vi "Log MBW Data.vi"() -> ()   [LabVIEW 2015]
uses:
  X Range.ctl
  MBW States.ctl
  <vilib>/Instr/_visa.llb/VISA Configure Serial Port (Instr).vi
  <vilib>/Utility/file.llb/Write To Spreadsheet File (string).vi
panel:
  out "Cycle Time, ms":u32=618
  out "Ch3":sgl=35854.33
  out "Ch2":sgl=35854.33
  out "Ch1":sgl=35854.33
  out "Ch0":sgl=26047.0
  in  "Re-Initialize":bool
  out "error out":errorcluster
  in  "States":T1=enum."Initialize"
  in  "CH D":u16(ring) items=["Time_s", "Stable", "Frostpoint_C", "DewPoint_C", "VolRatio_ppmv", "VaporPres_Pa", "HeadPres_Pa", "FlowRate_lpm", "MirrorT_C"]
  in  "CH C":u16(ring) items=["Time_s", "Stable", "Frostpoint_C", "DewPoint_C", "VolRatio_ppmv", "VaporPres_Pa", "HeadPres_Pa", "FlowRate_lpm", "MirrorT_C"]
  in  "CH B":u16(ring) items=["Time_s", "Stable", "Frostpoint_C", "DewPoint_C", "VolRatio_ppmv", "VaporPres_Pa", "HeadPres_Pa", "FlowRate_lpm", "MirrorT_C"]
  in  "CH A":u16(ring)=4 items=["Time_s", "Stable", "Frostpoint_C", "DewPoint_C", "VolRatio_ppmv", "VaporPres_Pa", "HeadPres_Pa", "FlowRate_lpm", "MirrorT_C"]
  out "Graph 2":sgl[][](graph)=[[35846.125, 35846.75, 35847.375, 35848.016, 35848.688, 35849.297, 35849.92, 35850.53, 35851.14, 35851.766, 35852.375, 35853.03, 35853.703], [35846.125, 35846.75, 35847.375, 35848.016, 35848.688, 35849.297, 35849.92, 35850.53, 35851.14, 35851.766, 35852.375, 35853.03, 35853.703]]
  out "Graph 1":sgl[][](graph)=[[25759.9, 25973.8, 25975.8, 25975.8, 25980.7, 25987.2, 25987.2, 25998.8, 25998.8, 26008.6, 26020.1, 26020.1, 26032.8], [35846.125, 35846.75, 35847.375, 35848.016, 35848.688, 35849.297, 35849.92, 35850.53, 35851.14, 35851.766, 35852.375, 35853.03, 35853.703]]
  in  "X Range":T2
  out "Current File":path=path "C:/MBW_Data/MBW20120124/MBW20120124x003.txt"
  in  "Base Path":path=path "C:/MBW_Data"
  in  "stop":bool
  in  "Column Header (comma del)":string="Time_s,Stable,Frostpoint_C,DewPoint_C,VolRatio_ppmv,VaporPres_Pa,HeadPres_Pa,FlowRate_lpm,MirrorT_C"
  in  "Sample rate (S)":u32=1
  in  "Commands to send":string[](array[string])=["Stable?", "FP?", "DP?", "PPMv?", "VP?", "P?", "Flow?", "Tm?"]
  in  "Com Port":refnum<visa-resource-name>="COM4"
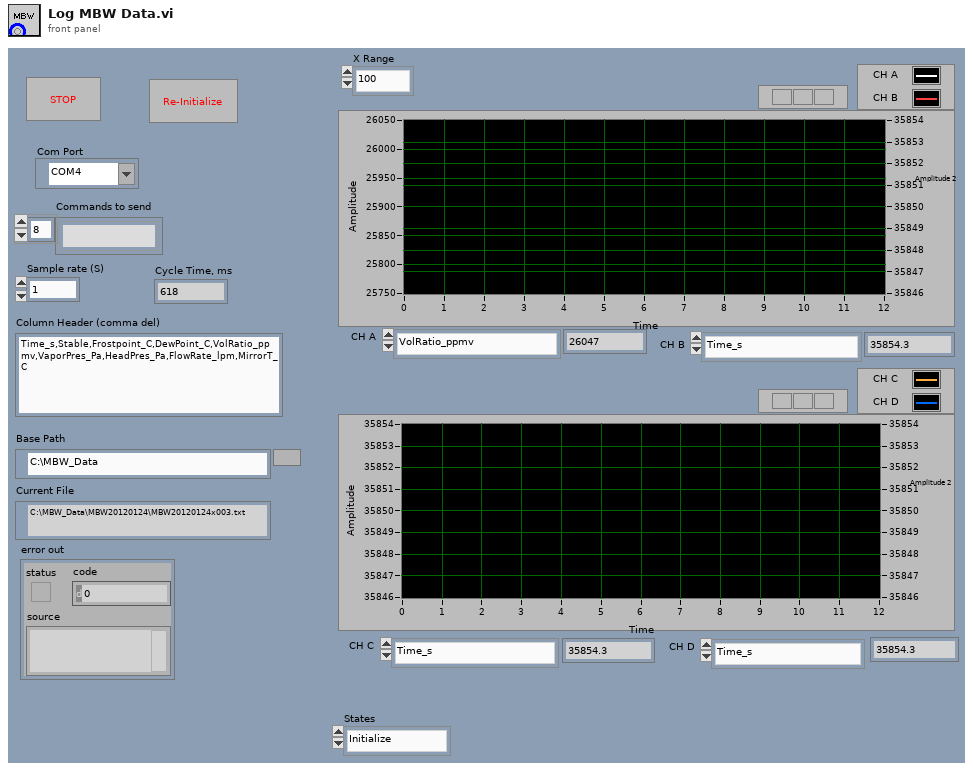
[diagram p1: front panel]
types:
  T1 = typedef "MBW States.ctl" = enum16{"Idle", "Initialize", "Check Buttons", "Send Commands", "Update Graph", "Write Data", "Close", "Exit"}
  T2 = typedef "X Range.ctl" = enum16{"100", "300", "500", "1000", "3000", "5000", "10000", "20000", "30000", "40000", "60000"}
  T3 = typedef "LVDateTimeRec.ctl" = cluster{"fractional second":dbl, "second":i32, "minute":i32, "hour":i32, "day of month":i32, "month":i32, "year":i32, "day of week":i32, "day of year":i32, "DST":i32}
  T4 = cluster{"CH A":u16, "CH B":u16, "CH C":u16, "CH D":u16}
  T5 = cluster{"Ch0":sgl, "Ch1":sgl, "Ch2":sgl, "Ch3":sgl}
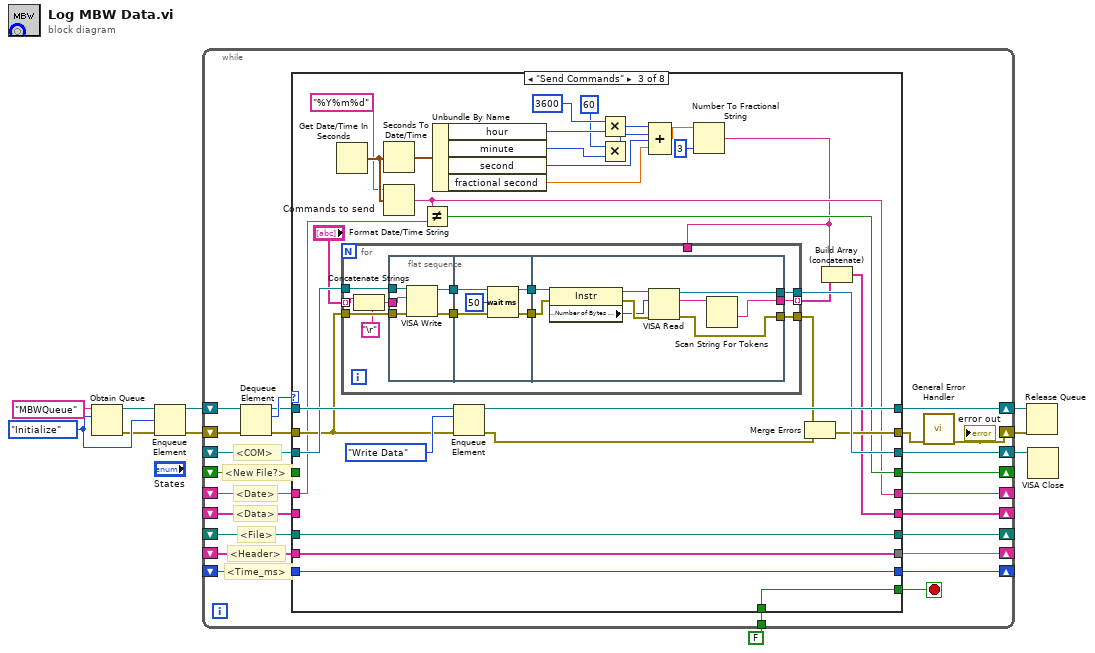
[diagram p0: block diagram]
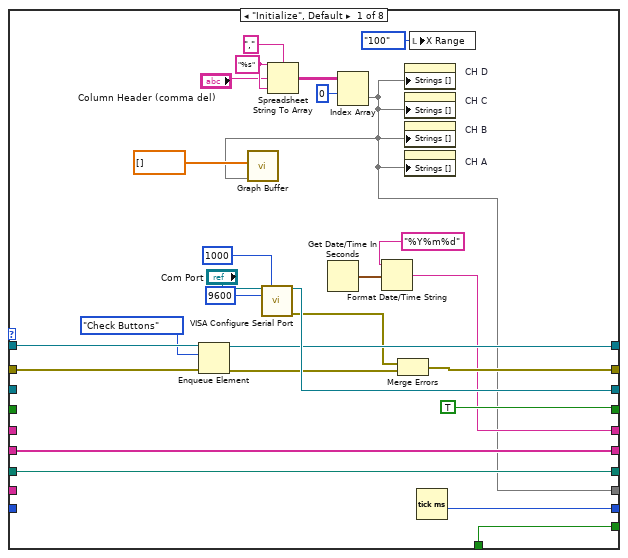
[diagram p2: hidden frame]
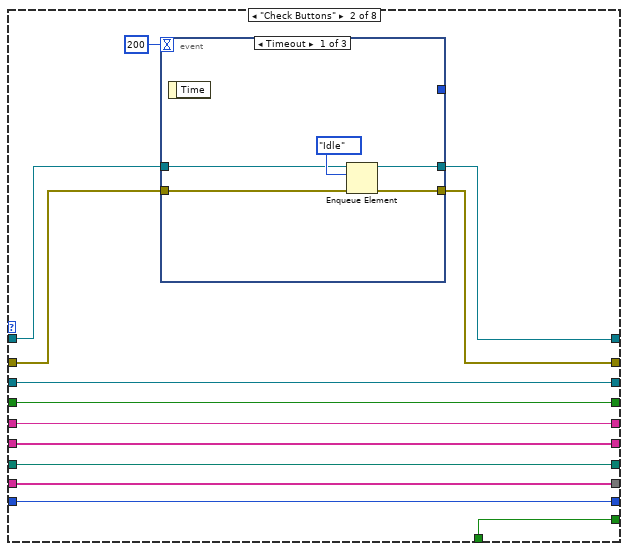
[diagram p3: hidden frame]
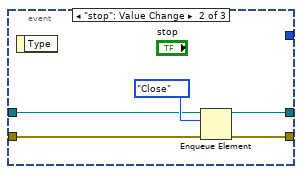
[diagram p4: hidden frame]
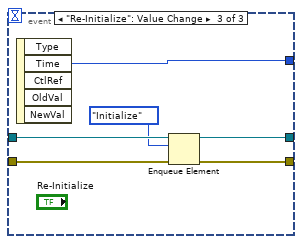
[diagram p5: hidden frame]
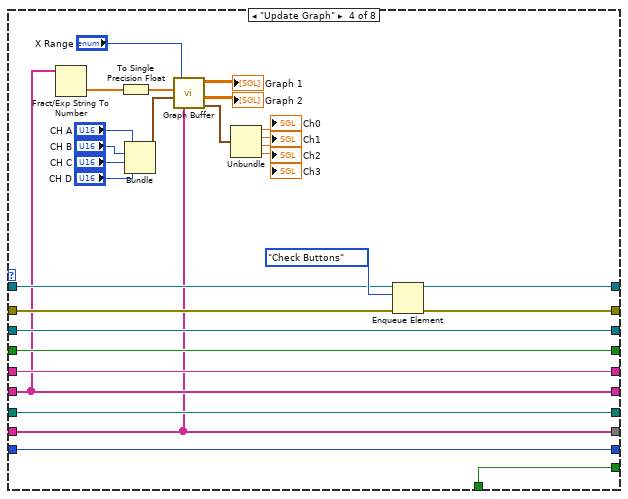
[diagram p6: hidden frame]
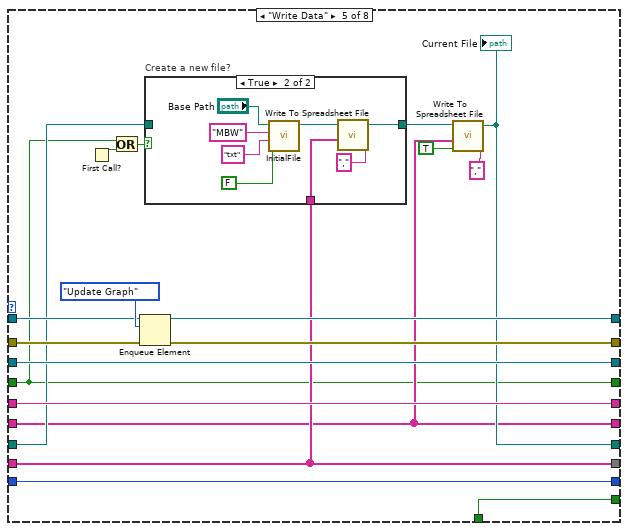
[diagram p7: hidden frame]
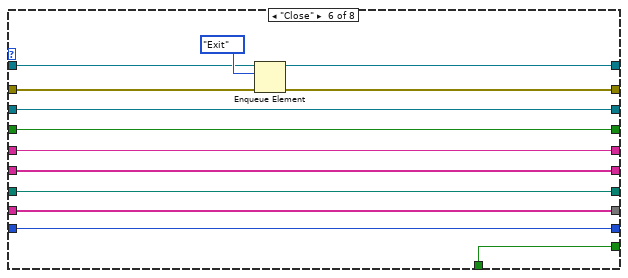
[diagram p9: hidden frame]
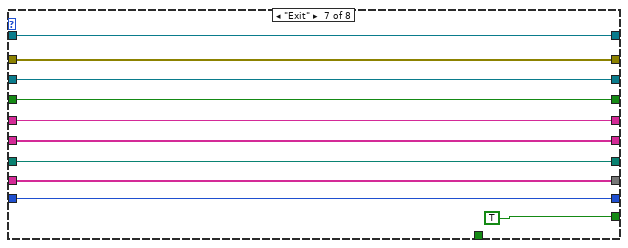
[diagram p10: hidden frame]
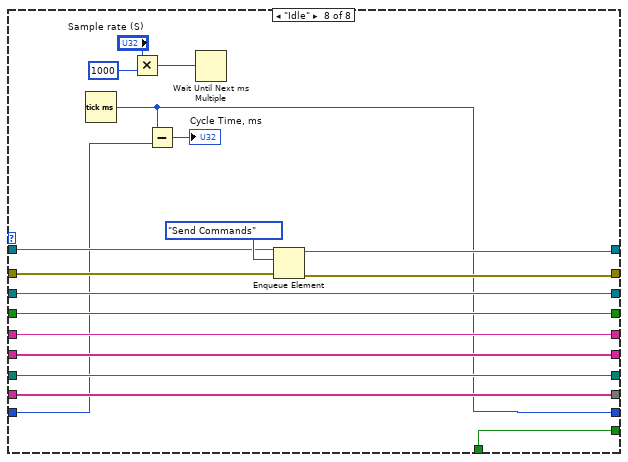
[diagram p11: hidden frame]
diagram:
  w9 = MBW_States."Initialize" ("States")
  n1 = Obtain Queue(name (unnamed)="MBWQueue", element data type=w9) -> (queue out=w8:refnum<queue>, error out=w7:errorcluster)  [unwired: 3 in, 1 out]
  n2 = Enqueue Element(queue=w8, element=w9, error in (no error)=w7) -> (queue out=w6:refnum<queue>, error out=w5:errorcluster)  [unwired: 1 in, 1 out]
  n3 = while {
    shift-right: [w25] -> w4
    shift-left: w6 -> [w28]
    shift-right: [w24] -> w3
    shift-left: w5 -> [w30]
    shift-right: [w33] -> w2
    shift-left: _ -> [w34]
    shift-right: [w31] -> _
    shift-left: _ -> [w32]
    shift-right: [w22] -> _
    shift-left: _ -> [w23]
    shift-right: [w20] -> _
    shift-left: _ -> [w21]
    shift-right: [w18] -> _
    shift-left: _ -> [w19]
    shift-right: [w16] -> _
    shift-left: _ -> [w17]
    tunnel: FALSE -> [w15]
    shift-right: [w12] -> _
    shift-left: _ -> [w13]
    stop <- w14 stop-if-true
    # "<Time_ms>"
    # "<Header>"
    # "<File>"
    # "<Date>"
    # "<Data>"
    # "<New File?>"
    # "<COM>"
    n4 = Dequeue Element(queue=w28, error in (no error)=w30) -> (queue out=w26:refnum<queue>, element=w27:T1, error out=w29:errorcluster)  [unwired: 1 in, 1 out]
    n5 = case shown="\"Send Commands\"" w27 {
      tunnel: w29 -> [w47 w71 w108 w174 w195 w211 w231 w236]
      tunnel: [w49 w68 w105 w173 w194 w210 w231 w237] -> w11
      tunnel: w34 -> [_ w74 w111 w180 w199 w221 w230 w249]
      tunnel: [w60 w74 w110 w180 w199 w221 w230 w249] -> w33
      tunnel: w32 -> [_ w73 _ w179 w183 w220 w229 w248]
      tunnel: [TRUE w73 w98 w179 w183 w220 w229 w248] -> w31
      tunnel: w26 -> [w48 w72 w122 w176 w197 w213 w228 w239]
      tunnel: [w52 w67 w121 w175 w196 w212 w228 w238] -> w25
      tunnel: w23 -> [_ w70 w99 w178 w193 w219 w227 w247]
      tunnel: [w41 w70 w97 w178 w193 w219 w227 w247] -> w22
      tunnel: w21 -> [w45 w69 _ w169 w188 w218 w226 w246]
      tunnel: [w45 w69 w101 w169 w188 w218 w226 w246] -> w20
      tunnel: w19 -> [w40 w66 w96 w172 w191 w217 w225 w245]
      tunnel: [w40 w66 w96 w172 w189 w217 w225 w245] -> w18
      tunnel: w17 -> [_ w65 w95 w161 w190 w216 w224 w244]
      tunnel: [w35 w65 w95 w161 w190 w216 w224 w244] -> w16
      tunnel: w15 -> [w39 w64 w94 w171 w186 w215 _ w243]
      tunnel: [w39 w64 w94 w171 w186 w215 TRUE w243] -> w14
      tunnel: w13 -> [_ w62 w92 w170 w185 w209 w222 w234]
      tunnel: [w38 w62 w92 w170 w185 w209 w222 w233] -> w12
      frame "Initialize", Default {
        w58 = "%s" ("format string")
        n6 = Enqueue Element(queue=w48, element=MBW_States."Check Buttons", error in (no error)=w47) -> (queue out=w52:refnum<queue>, error out=w50:errorcluster)  [unwired: 1 in, 1 out]
        n7 = call-poly "VISA Configure Serial Port"("VISA resource name"="Com Port", "timeout (10sec)"=u32 1000, "baud rate (9600)"=u32 9600) -> ("VISA resource name out"=w60:refnum<visa-resource-name>, "error out"=w51:errorcluster)  [unwired: 11 in]
        n8 = Spreadsheet String To Array(delimiter (Tab)=",", format string=w58, spreadsheet string="Column Header (comma del)", array type (2D Dbl)=w58) -> (array=w36:string[][])
        n9 = Get Date/Time In Seconds() -> (seconds since 1Jan1904=w42:timestamp)
        n10 = Index Array(array=w36, index (row)=0) -> (element=w35:string[])  [unwired: 1 in]
        n11 = call "Graph Buffer.vi"("Channel Names"=w35, "Data"=sgl[] []) -> ()  [unwired: 3 in, 3 out]
        n12 = Format Date/Time String(time format string (%c)="%Y%m%d", seconds (now)=w42) -> (date/time string=w41:string)  [unwired: 1 in]
        n13 = Merge Errors(w51, w50) -> (w49:errorcluster)
        n14 = property on="CH D" class="Ring (strict)"("Strings []"=w35) -> ()  [unwired: 2 in, 2 out]
        n15 = property on="CH C" class="Ring (strict)"("Strings []"=w35) -> ()  [unwired: 2 in, 2 out]
        n16 = property on="CH B" class="Ring (strict)"("Strings []"=w35) -> ()  [unwired: 2 in, 2 out]
        n17 = property on="CH A" class="Ring (strict)"("Strings []"=w35) -> ()  [unwired: 2 in, 2 out]
        n18 = local write "X Range"(X_Range."100" ("X Range")) -> ()
        n19 = Tick Count (ms)() -> (millisecond timer value=w38:u32)
      }
      frame "Check Buttons" {
        n20 = event shown="[0] Timeout" {
          selector: _ -> [_ _ _]
          dyn-events: _ -> [_ _ _]
          timeout: 200 -> [_ _ _]
          tunnel: w72 -> [w76 w83 w90]
          tunnel: w71 -> [w75 w81 w89]
          tunnel: [w77 w80 w88] -> w68
          tunnel: [w78 w82 w87] -> w67
          tunnel: [_ _ w85] -> _
          event Timeout {
            n21 = event-data() -> ()  [unwired: 1 in, 1 out]
            n22 = Enqueue Element(queue=w76, element=MBW_States."Idle", error in (no error)=w75) -> (queue out=w78:refnum<queue>, error out=w77:errorcluster)  [unwired: 1 in, 1 out]
          }
          event "stop": Value Change {
            n23 = event-data() -> ()  [unwired: 1 in, 1 out]
            n24 = Enqueue Element(queue=w83, element=MBW_States."Close", error in (no error)=w81) -> (queue out=w82:refnum<queue>, error out=w80:errorcluster)  [unwired: 1 in, 1 out]
          }
          event "Re-Initialize": Value Change {
            n25 = event-data() -> ("Time"=w85:u32)  [unwired: 1 in, 4 out]
            n26 = Enqueue Element(queue=w90, element=MBW_States."Initialize", error in (no error)=w89) -> (queue out=w87:refnum<queue>, error out=w88:errorcluster)  [unwired: 1 in, 1 out]
          }
        }
      }
      frame "Send Commands" {
        n27 = Get Date/Time In Seconds() -> (seconds since 1Jan1904=w100:timestamp)
        n28 = Seconds To Date/Time(time stamp (now)=w100) -> (date time rec=w120:T3)  [unwired: 1 in]
        n29 = Format Date/Time String(time format string (%c)="%Y%m%d", seconds (now)=w100) -> (date/time string=w97:string)  [unwired: 1 in]
        n30 = Not Equal?(x=w97, y=w99) -> (x != y?=w98:bool)
        n31 = Unbundle By Name(w120) -> ("hour"=w119:i32, "minute"=w117:i32, "second"=w113:i32, "fractional second"=w112:dbl)
        n32 = Enqueue Element(queue=w122, element=MBW_States."Write Data", error in (no error)=w108) -> (queue out=w121:refnum<queue>, error out=w107:errorcluster)  [unwired: 1 in, 1 out]
        n33 = Multiply(x=3600, y=w119) -> (x*y=w115:i32)
        n34 = Multiply(x=60, y=w117) -> (x*y=w114:i32)
        n35 = Compound Arithmetic op=ADD(w115, w114, w113, w112) -> (w104:dbl)
        n36 = Number To Fractional String(number=w104, precision (6)=i16 3) -> (F-format string=w93:string)  [unwired: 2 in]
        n37 = for {
          tunnel: w111 -> [w135]
          tunnel: [w132] -> w110
          tunnel: "Commands to send" -> [w126] mode=indexing
          tunnel: [w129] -> w106
          tunnel: w108 -> [w128]
          tunnel: [w127] -> w102 mode=indexing
          tunnel: w93 -> [_]
          n38 = Concatenate Strings(w126, "\r") -> (w125:string)
          n39 = flat-sequence {
            tunnel: w135 -> [w140]
            tunnel: [w139] -> w133
            tunnel: w125 -> [w138]
            tunnel: [w137] -> w130
            tunnel: w128 -> [w136]
            tunnel: [w143] -> w134
            tunnel: w133 -> [w143]
            tunnel: [w142] -> w131
            tunnel: w130 -> [w142]
            tunnel: w134 -> [w152]
            tunnel: [w150] -> w132
            tunnel: w131 -> [w149]
            tunnel: [w144] -> w129
            tunnel: [w145] -> w127
            frame #0 {
              n40 = VISA Write(VISA resource name=w140, write buffer=w138, error in (no error)=w136) -> (VISA resource name out=w139:refnum<visa-resource-name>, error out=w137:errorcluster)  [unwired: 1 out]
            }
            frame #1 {
              n41 = Wait (ms)(milliseconds to wait=u32 50) -> ()  [unwired: 1 out]
            }
            frame #2 {
              n42 = property class="Instr"(reference=w152, error in=w149) -> (reference out=w151:refnum<visa-resource-name>, error out=w148:errorcluster, "Serial Settings:Number of Bytes at Serial Port"=w147:u32)
              n43 = VISA Read(VISA resource name=w151, byte count=w147, error in (no error)=w148) -> (VISA resource name out=w150:refnum<visa-resource-name>, read buffer=w146:string, error out=w144:errorcluster)  [unwired: 1 out]
              n44 = Scan String For Tokens(9:w146) -> (1:w145:string)  [unwired: 5 in, 3 out]
            }
          }
        }
        n45 = Merge Errors(w106, w107) -> (w105:errorcluster)
        n46 = Build Array (concatenate)(w93, w102) -> (w101:string[])
      }
      frame "Update Graph" {
        n47 = Fract/Exp String To Number(string=w169) -> (number=w168:dbl[])  [unwired: 3 in, 1 out]
        n48 = To Single Precision Float(number=w168) -> (single precision float=w153:sgl[])
        n49 = Bundle("CH A"="CH A", "CH B"="CH B", "CH C"="CH C", "CH D"="CH D") -> (w162:T4)  [unwired: 1 in]
        n50 = call "Graph Buffer.vi"("Channel Names"=w161, "Channels"=w162, "Data"=w153, "X Range"="X Range") -> ("LastValues"=w158:T5, "Graph 2"=→"Graph 2":sgl[][], "Graph 1"=→"Graph 1":sgl[][])  [unwired: 1 in]
        n51 = Unbundle(w158) -> ("Ch0"=→"Ch0":sgl, "Ch1"=→"Ch1":sgl, "Ch2"=→"Ch2":sgl, "Ch3"=→"Ch3":sgl)
        n52 = Enqueue Element(queue=w176, element=MBW_States."Check Buttons", error in (no error)=w174) -> (queue out=w175:refnum<queue>, error out=w173:errorcluster)  [unwired: 1 in, 1 out]
      }
      frame "Write Data" {
        n53 = First Call?() -> (First Call?: T/F=w182:bool)
        n54 = Or(x=w183, y=w182) -> (x .or. y?=w181:bool)
        n55 = Enqueue Element(queue=w197, element=MBW_States."Update Graph", error in (no error)=w195) -> (queue out=w196:refnum<queue>, error out=w194:errorcluster)  [unwired: 1 in, 1 out]
        n56 = case "Create a new file?" shown="True" w181 {
          tunnel: [w200 w204] -> w192
          tunnel: w191 -> [w200 _]
          tunnel: w190 -> [_ w202]
          frame False {
          }
          frame True {
            n57 = call "InitialFile.vi"("UTC format"=FALSE, "Extension"="txt", "PreAppend Name"="MBW", "Base Path"="Base Path") -> ("File Path"=w203:path)  [unwired: 7 in]
            n58 = call-poly <vilib>:"Write To Spreadsheet File.vi"("delimiter (\\t)"="," ("delimiter (\\t)"), "1D data"=w202, "file path (dialog if empty)"=w203) -> ("new file path (Not A Path if cancelled)"=w204:path)  [unwired: 5 in]
          }
        }
        n59 = call-poly <vilib>:"Write To Spreadsheet File.vi"("delimiter (\\t)"="," ("delimiter (\\t)"), "append to file? (new file:F)"=TRUE, "1D data"=w188, "file path (dialog if empty)"=w192) -> ("new file path (Not A Path if cancelled)"=w189:path)  [unwired: 4 in]
        "Current File" <- w189
      }
      frame "Close" {
        n60 = Enqueue Element(queue=w213, element=MBW_States."Exit", error in (no error)=w211) -> (queue out=w212:refnum<queue>, error out=w210:errorcluster)  [unwired: 1 in, 1 out]
      }
      frame "Exit" {
      }
      frame "Idle" {
        n61 = Tick Count (ms)() -> (millisecond timer value=w233:u32)
        n62 = Multiply(x="Sample rate (S)", y=u32 1000) -> (x*y=w235:u32)
        n63 = Subtract(x=w233, y=w234) -> (x-y=→"Cycle Time, ms":u32)
        n64 = Wait Until Next ms Multiple(millisecond multiple=w235) -> ()  [unwired: 1 out]
        n65 = Enqueue Element(queue=w239, element=MBW_States."Send Commands", error in (no error)=w236) -> (queue out=w238:refnum<queue>, error out=w237:errorcluster)  [unwired: 1 in, 1 out]
      }
    }
    n66 = call <vilib>:"General Error Handler.vi"("error in (no error)"=w11) -> ("error out"=w24:errorcluster)  [unwired: 10 in, 4 out]
    "error out" <- w24
  }
  n67 = Release Queue(queue=w4, error in (no error)=w3) -> ()  [unwired: 1 in, 3 out]
  n68 = VISA Close(VISA resource name=w2) -> ()  [unwired: 1 in, 1 out]
